vi "BMark_Choose Bookmark Manager Dialog.vi"(10 "previously selected":i32 caption="以前选中", 11 "Item names":string[](array[string]) caption="项名") -> (1 "do not show":bool caption="不再显示", 2 "Selected bookmark manager":i32 caption="选中的书签管理器", 3 "Cancelled?":bool caption="取消？")   [LabVIEW 2016]
panel:
  in  "Select a Bookmark Manager":i32(listbox) caption="选择书签管理器"
  in  "Do not show again":bool caption="下次不再显示"
  in  "Help":bool caption="帮助"
  in  "Cancel":bool caption="取消"
  in  "OK":bool caption="确定"
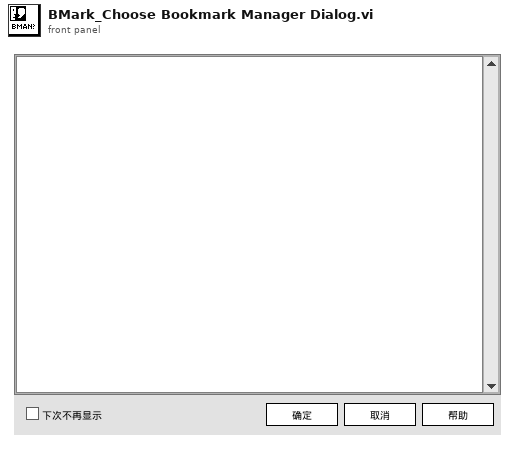
[diagram p1: front panel]
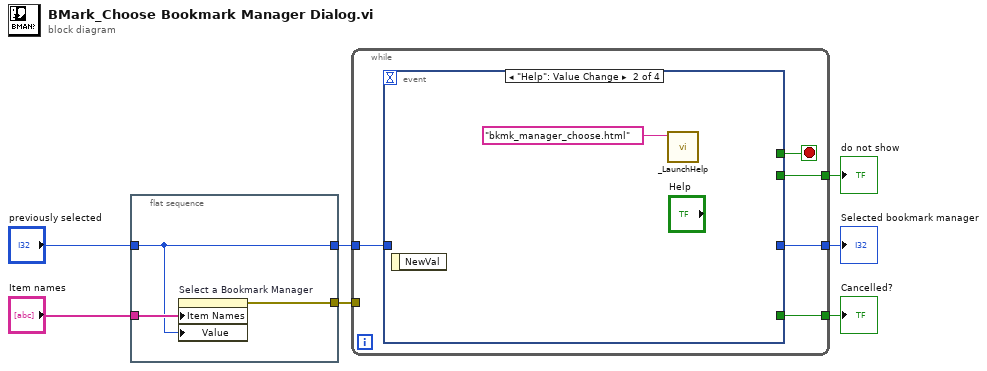
[diagram p0: block diagram]
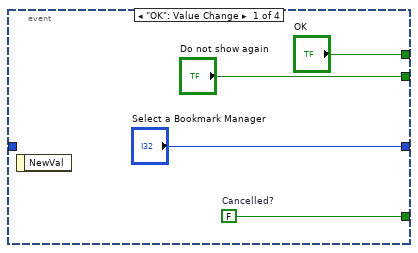
[diagram p2: hidden frame]
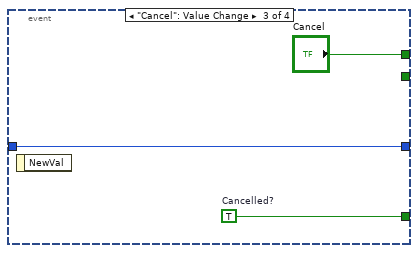
[diagram p3: hidden frame]
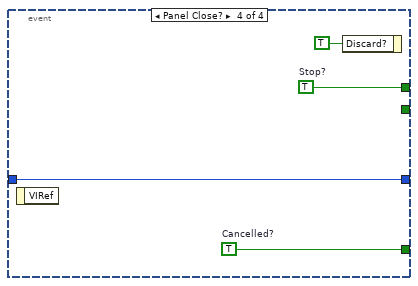
[diagram p4: hidden frame]
diagram:
  n1 = flat-sequence {
    tunnel: "Item names" -> [w10]
    tunnel: [w9] -> w4
    tunnel: "previously selected" -> [w8]
    tunnel: [w8] -> w1
    frame #0 {
      n2 = property on="Select a Bookmark Manager" class="LstBox (strict)"("Item Names"=w10, "Value"=w8) -> (error out=w9:errorcluster)  [unwired: 2 in, 1 out]
    }
  }
  n3 = while {
    tunnel: [w14] -> w7
    tunnel: [w13] -> w6
    tunnel: w4 -> [_]
    tunnel: [w12] -> w3
    tunnel: w1 -> [w11]
    stop <- w15 stop-if-true
    n4 = event shown="[1] \"Help\": Value Change" {
      selector: _ -> [_ _ _ _]
      dyn-events: _ -> [_ _ _ _]
      timeout: _ -> [_ _ _ _]
      tunnel: ["OK" _ "Cancel" w26] -> w15
      tunnel: [w19 _ w23 w25] -> w14
      tunnel: ["Select a Bookmark Manager" _ w21 w24] -> w13
      tunnel: ["Do not show again" _ _ _] -> w12
      tunnel: w11 -> [_ _ w21 w24]
      event "OK": Value Change {
        w19 = FALSE  # Cancelled?
        n5 = event-data() -> ()  [unwired: 1 in, 1 out]
      }
      event "Help": Value Change {
        n6 = event-data() -> ()  [unwired: 1 in, 1 out]
        n7 = call <helpdir>:"_LaunchHelp.vi"("HTML filename"="bkmk_manager_choose.html") -> ()  [unwired: 6 in, 1 out]
      }
      event "Cancel": Value Change {
        w23 = TRUE  # Cancelled?
        n8 = event-data() -> ()  [unwired: 1 in, 1 out]
      }
      event Panel Close? {
        w25 = TRUE  # Cancelled?
        w26 = TRUE  # Stop?
        n9 = event-data() -> ()  [unwired: 1 in, 1 out]
        n10 = event-data("Discard?"=TRUE) -> ()  [unwired: 1 in, 1 out]
      }
    }
  }
  "Cancelled?" <- w7
  "Selected bookmark manager" <- w6
  "do not show" <- w3
